vi "dmx.vi"(1 "CONTROL":T1, 2 "INPUT":T2) -> (0 "OUTPUT":T3)   [LabVIEW 2013]
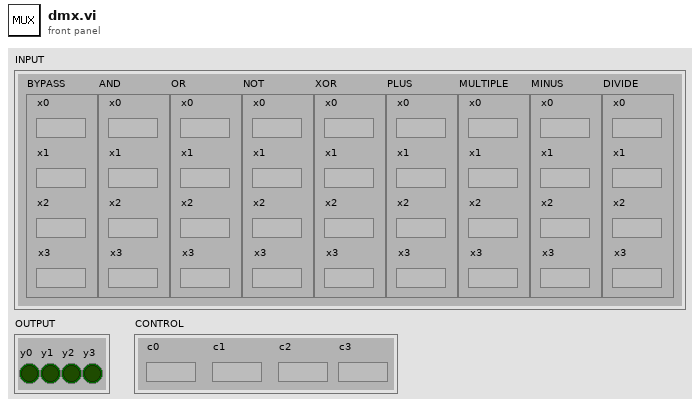
[diagram p1: front panel]
types:
  T1 = cluster{"c0":bool, "c1":bool, "c2":bool, "c3":bool}
  T2 = cluster{"BYPASS":cluster{"x0":bool, "x1":bool, "x2":bool, "x3":bool}, "AND":cluster{"x0":bool, "x1":bool, "x2":bool, "x3":bool}, "OR":cluster{"x0":bool, "x1":bool, "x2":bool, "x3":bool}, "NOT":cluster{"x0":bool, "x1":bool, "x2":bool, "x3":bool}, "XOR":cluster{"x0":bool, "x1":bool, "x2":bool, "x3":bool}, "PLUS":cluster{"x0":bool, "x1":bool, "x2":bool, "x3":bool}, "MULTIPLE":cluster{"x0":bool, "x1":bool, "x2":bool, "x3":bool}, "MINUS":cluster{"x0":bool, "x1":bool, "x2":bool, "x3":bool}, "DIVIDE":cluster{"x0":bool, "x1":bool, "x2":bool, "x3":bool}}
  T3 = cluster{"y0":bool, "y1":bool, "y2":bool, "y3":bool}
  T4 = cluster{"x0":bool, "x1":bool, "x2":bool, "x3":bool}
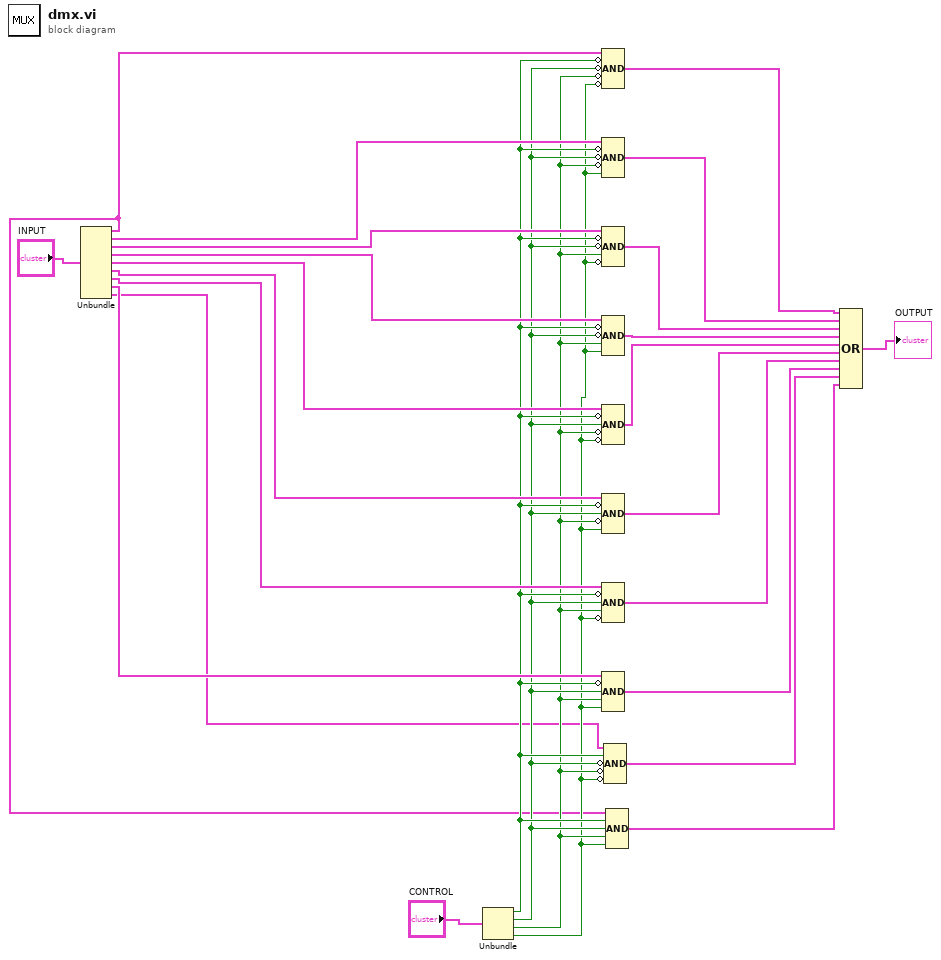
[diagram p0: block diagram]
diagram:
  n1 = Unbundle("INPUT") -> ("BYPASS"=w1:T4, "AND"=w25:T4, "OR"=w24:T4, "NOT"=w23:T4, "XOR"=w22:T4, "PLUS"=w21:T4, "MULTIPLE"=w20:T4, "MINUS"=w19:T4, "DIVIDE"=w2:T4)
  n2 = Unbundle("CONTROL") -> ("c0"=w6:bool, "c1"=w5:bool, "c2"=w4:bool, "c3"=w3:bool)
  n3 = Compound Arithmetic op=AND(w1, invert w6, invert w5, invert w4, invert w3) -> (w16:T4)
  n4 = Compound Arithmetic op=AND(w25, invert w6, invert w5, invert w4, w3) -> (w15:T4)
  n5 = Compound Arithmetic op=AND(w24, invert w6, invert w5, w4, invert w3) -> (w14:T4)
  n6 = Compound Arithmetic op=AND(w23, invert w6, invert w5, w4, w3) -> (w13:T4)
  n7 = Compound Arithmetic op=AND(w22, invert w6, w5, invert w4, invert w3) -> (w12:T4)
  n8 = Compound Arithmetic op=AND(w21, invert w6, w5, invert w4, w3) -> (w11:T4)
  n9 = Compound Arithmetic op=AND(w20, invert w6, w5, w4, invert w3) -> (w10:T4)
  n10 = Compound Arithmetic op=AND(w19, invert w6, w5, w4, w3) -> (w9:T4)
  n11 = Compound Arithmetic op=AND(w2, w6, invert w5, invert w4, invert w3) -> (w7:T4)
  n12 = Compound Arithmetic op=AND(w1, w6, w5, w4, w3) -> (w8:T4)
  n13 = Compound Arithmetic op=OR(w16, w15, w14, w13, w12, w11, w10, w9, w7, w8) -> (→"OUTPUT":T4)
